vi "OFDM_demo.vi"() -> ()   [LabVIEW 2009]
uses:
  <vilib>/imath/engines/lvmath2/RunTimeEngine/ErrorHandling/NIMS_Finalize Error.vi
  <vilib>/imath/engines/lvmath2/RunTimeEngine/Parser/MC_Version.vi
  <vilib>/imath/engines/lvmath2/RunTimeEngine/NodeEndStatement/NIMS_NodeEndStatement_Output.vi
  <instcachedir>/0/NIMS_NodeEndStatement_Output_53EC0D466D134D7ABD903AC30B43404B.lvgen/NIMS_NodeEndStatement_Output_53EC0D466D134D7ABD903AC30B43404B_001.vi
  <vilib>/imath/engines/lvmath2/RunTimeEngine/RangeToken/NIMS_Range.vi
  <instcachedir>/0/NIMS_Range_08574DECC23E450FAF0AC0BC39E6BEA7.lvgen/NIMS_Range_08574DECC23E450FAF0AC0BC39E6BEA7_000.vi
  <vilib>/imath/engines/lvmath2/RunTimeEngine/BuiltInFunctions/round/NIMS_round(DBL-S).vi
  <vilib>/imathl/engines/lvmath/Functions/Error Handling/Create Error.vi
  <vilib>/imath/engines/lvmath/Functions/Error Handling/MC_Error Cluster From Error Code.vi
  <vilib>/imath/engines/lvmath2/RunTimeEngine/BuiltInFunctions/randnormal/NIMS_randnormal(1,I32).vi
  <vilib>/imath/engines/lvmath2/RunTimeEngine/RangeToken/NIMS_Range_R2 - Float.vi
  <instcachedir>/0/NIMS_Range_R2 - Float_93A1434467634702BCAD427B3499A8B4.lvgen/NIMS_Range_R2 - Float_93A1434467634702BCAD427B3499A8B4_000.vi
  <vilib>/imath/engines/lvmath/Functions/Error Handling/MergeErrorsWrapper.vi
  <vilib>/imath/engines/lvmath2/RunTimeEngine/ArithmeticOperatorToken/NIMS_ArithmeticOperator_plus.vi
  <instcachedir>/0/NIMS_ArithmeticOperator_plus_48B9519178ED42D7840F01273E784BFE.lvgen/NIMS_ArithmeticOperator_plus_48B9519178ED42D7840F01273E784BFE_000.vi
  <vilib>/imath/engines/lvmath2/RunTimeEngine/CommandStatement/MC_CommandStatement_break.vi
  <vilib>/imath/engines/lvmath2/RunTimeEngine/BuiltInFunctions/abs/NIMS_abs(signed).vi
  <instcachedir>/0/NIMS_abs(signed)_C4FCB8E6058B49B797C7C8D53CA5F6EC.lvgen/NIMS_abs(signed)_C4FCB8E6058B49B797C7C8D53CA5F6EC_000.vi
  <vilib>/imath/engines/lvmath2/RunTimeEngine/BuiltInFunctions/fft/NIMS_fft(GV).vi
  <instcachedir>/0/NIMS_fft(GV)_4C6467FC22F84E4BA42517A07EF978B0.lvgen/NIMS_fft(GV)_4C6467FC22F84E4BA42517A07EF978B0_001.vi
panel:
  in  "Number of Signals":dbl
  out "Frequency Domain":dbl[](graph)=[-65.85915777379863, -67.4159182508014, -83.98237928756325, -67.68454807939689, 0.001167659462857509, -62.00279471774978, -76.50031843632243, -79.84930333750974, -0.002321301830740114, -70.28161681379156, -75.37014688475936, -71.43223279356836, 0.0019758076165627735, -67.19023864671585, -59.326071900571705, -71.57758360782793, -0.0033451837990704854, -64.73231439603472, -68.3545781993946, -64.47936727351482, -0.004934079437755126, -63.18690880959889, -76.85128578370852, -77.1128911079366, -0.0015364990671404202, -60.09670538205802, -70.0061247105409, -66.3416220582635, 0.00308476690655415, -65.11673413833363, -69.99982685419918, -70.73910551220207, -0.0003146063843862787, -74.23065363786773, -82.56015032934161, -73.17243303091855, -0.005390191213401431, -64.32159403220355, -71.98817626923424, -69.2227375887466, -0.0025172993098405987, -66.25303750066834, -71.07288503298095, -68.5714475641465, -0.0026506959056577543, -72.79019967143984, -67.38892881214208, -63.8704912590564, 0.00015780098831987704, -68.67653217007089, -64.72051278103325, -64.4623299664106, 0.002984864272674666, -68.607590443405, -63.48155974398481, -66.18996423364395, -0.0027916165109335765, -63.627998158951996, -66.10830696818293, -71.77885901545312, -0.005305794062812742, -68.5330696250455, -65.18053285890313, -75.28656898448178, -0.0012317224408319144, -66.48761574232225, -65.79637197270438, -66.5523728488871, -0.002458779881879369, -64.93250339047772, -66.95401625552422, -72.71143622458413, -0.003663998535422267, -74.4964256353411, -71.53601578586682, -72.10926464858508, -0.0033669659636299397, -81.08779383955226, -69.63851872055983, -66.00644993381869, 0.002853851739313183, -65.03887110061628, -71.65894945859802, -68.7667431871805, 0.001286174703623317, -64.82909545506283, -67.84252983844794, -64.00457445122368, -0.0005370860401690884, -68.57259285794203, -73.0607979439583, -67.38041679413246, -0.000819699000330847, -71.11688188519892, -79.12328832965329, -74.4243659108799, -0.003680712718152329, -66.39506517793357, -72.10292803376697, -73.75934014796238, -0.0012648503306429636, -75.48974485549587, -67.35819567344844, -66.29114964266908, 0.0011096917850492642, -75.78825076994536, -68.6498880937598, -73.89622602097464, 0.00450716809119083, -70.98318173363074, -71.3103499892423, -73.81175836011673, -0.001276663889058421, -64.46629884383417, -74.36488154213885, -67.93429426887408, 0.0033684081216353097, -77.79388616517662, -66.26157587608216, -72.76220739766408, -0.0005132127073009369, -70.04594038061202, -73.19573222166245, -67.47769079029007, 0.0005524955358213877, -77.54300550351729, -71.04328528942425, -76.2420773706609, 6.0177378814099844, -76.2420773706609, -71.04328528942425, -77.54300550351729, 0.0005524955358213877, -67.47769079029007, -73.19573222166245, -70.04594038061202, -0.0005132127073009369, -72.76220739766408, -66.26157587608216, -77.79388616517662, 0.0033684081216353097, -67.93429426887408, -74.36488154213885, -64.46629884383417, -0.001276663889058421, -73.81175836011673, -71.3103499892423, -70.98318173363074, 0.00450716809119083, -73.89622602097464, -68.6498880937598, -75.78825076994536, 0.0011096917850492642, -66.29114964266908, -67.35819567344844, -75.48974485549587, -0.0012648503306429636, -73.75934014796238, -72.10292803376697, -66.39506517793357, -0.003680712718152329, -74.4243659108799, -79.12328832965329, -71.11688188519892, -0.000819699000330847, -67.38041679413246, -73.0607979439583, -68.57259285794203, -0.0005370860401690884, -64.00457445122368, -67.84252983844794, -64.82909545506283, 0.001286174703623317, -68.7667431871805, -71.65894945859802, -65.03887110061628, 0.002853851739313183, -66.00644993381869, -69.63851872055983, -81.08779383955226, -0.0033669659636299397, -72.10926464858508, -71.53601578586682, -74.4964256353411, -0.003663998535422267, -72.71143622458413, -66.95401625552422, -64.93250339047772, -0.002458779881879369, -66.5523728488871, -65.79637197270438, -66.48761574232225, -0.0012317224408319144, -75.28656898448178, -65.18053285890313, -68.5330696250455, -0.005305794062812742, -71.77885901545312, -66.10830696818293, -63.627998158951996, -0.0027916165109335765, -66.18996423364395, -63.48155974398481, -68.607590443405, 0.002984864272674666, -64.4623299664106, -64.72051278103325, -68.67653217007089, 0.00015780098831987704, -63.8704912590564, -67.38892881214208, -72.79019967143984, -0.0026506959056577543, -68.5714475641465, -71.07288503298095, -66.25303750066834, -0.0025172993098405987, -69.2227375887466, -71.98817626923424, -64.32159403220355, -0.005390191213401431, -73.17243303091855, -82.56015032934161, -74.23065363786773, -0.0003146063843862787, -70.73910551220207, -69.99982685419918, -65.11673413833363, 0.00308476690655415, -66.3416220582635, -70.0061247105409, -60.09670538205802, -0.0015364990671404202, -77.1128911079366, -76.85128578370852, -63.18690880959889, -0.004934079437755126, -64.47936727351482, -68.3545781993946, -64.73231439603472, -0.0033451837990704854, -71.57758360782793, -59.326071900571705, -67.19023864671585, 0.0019758076165627735, -71.43223279356836, -75.37014688475936, -70.28161681379156, -0.002321301830740114, -79.84930333750974, -76.50031843632243, -62.00279471774978, 0.001167659462857509, -67.68454807939689, -83.98237928756325, -67.4159182508014]
  out "Time Domain":dbl[](graph)=[32.00017112657278, -0.9983639293211752, 0.0008735355765997774, -1.0006091864923676, -0.0008656869615855403, -1.0002335780936629, -0.00012129659837191426, -1.0001721698210528, -0.005885422759168148, -0.995466661227796, -0.004419503619924629, -0.9948777723809261, 0.009332716893097842, -1.0031621642565403, -0.005016797304348691, -0.9964860889351613, -0.0021928490793982924, -1.0024576825906244, -0.006738884366811255, -0.9987835275908614, 0.0039564770633647, -1.0003854961966576, 6.529678604641038e-06, -0.9970424913742466, 0.003502863458182443, -1.000692082391001, 0.0016250124608794567, -0.99422494631012, 0.003640914889297361, -0.9998432185664662, -0.0005447667660256039, -0.996443898165778, 0.0003257808711581042, -0.9996152464607571, -0.002224165093202351, -0.9978196895746773, -0.006961344911486943, -1.0056132621276692, 0.0035615820280402053, -0.9984954841944591, 0.0023471787616144947, -1.0003846450004907, 0.0003302196259483037, -0.9990707669254306, 0.0036869433448601186, -0.9959639631261131, -0.0024015922345509873, -0.9990241319338568, -0.0014280381465069918, -0.9992900557634233, -0.0006415258476339477, -1.0039434357240529, -0.003933601587931967, -1.0019313163574013, 0.0005454145473986448, -1.0018604304189782, 0.00403129748804911, -0.995437793641305, -0.005078931896044563, -1.0004495062228045, -0.005667783175749135, -0.9950542453227285, -0.0010337477168682106, -1.0022702517624842, 31.996027861003995, -0.9992514696156752, 0.0023767417816136084, -0.9997573290965603, -0.00039079003427221735, -0.9972134852336257, 0.005253686163457493, -1.0019939747139937, -0.004615533899253865, -0.9999051627019617, 0.00174799695255463, -1.0008786334695843, 0.001040669585266476, -1.005631026866133, -0.00547826317021149, -1.0023984346670276, -0.0027209500680011023, -0.996926210417798, 0.004245827029374424, -0.9908809690660855, 0.0012736112257591991, -0.9983506650129511, -0.0024325566434215723, -1.0006700170865472, 0.003758930557249231, -1.0008199390652954, -0.00495900637739975, -1.003195189844263, -0.003449946260355973, -1.0008844588828651, -0.004112811651621141, -0.9995692117684838, 0.00039901886682617096, -1.000092063923351, 0.0021904132853824945, -0.9996356218624468, -0.0031081899271052653, -0.9991290221268253, 0.0027814082328749845, -1.0042300825504513, 0.0007163755121893314, -1.0013738837926813, -0.002538792067750837, -0.9997340068007473, 0.0031145063355714833, -1.00265950628907, -0.0004994034431624302, -0.9953760542096003, -0.002220859056506546, -1.0028537088428187, -0.0012009398756833648, -0.9963876808995135, 0.004768760241834631, -0.9988748054848854, 0.0004629995822051019, -0.9931078961670632, 0.002545476360266715, -1.0019962837613938, -0.0022606422179376326, -0.9955786638603721, -0.0006924783241974094, -1.0028097946283656, 0.0022509910529535946, -1.0043067841099833, 31.99308003375583, -1.0001975340020772, 0.0021521854173844873, -0.9964118152399534, 0.003451367454775092, -0.9982888588698008, 0.006709484384478659, -0.9943155486316583, 0.0023814148373482464, -0.9979859342389567, 0.002235599312541466, -1.0029388948536755, -0.0020749778600156654, -1.0046658275230822, -0.0076258112996254925, -0.9963324978398147, 0.007018563793711626, -0.9988749930014421, 0.00419471946131488, -0.997885450006954, -0.000586527863609928, -1.0024712482193048, -0.00031637483178920025, -1.0025777139206555, -0.001953463813398981, -1.0035333596290277, 0.0023257692492336048, -1.001220034251286, 0.001257832921962865, -1.0066843368331628, -0.004167328879506316, -0.9968152695189401, -0.004023488352167673, -1.0010141187149342, -0.007793457377208724, -0.9939375030812706, 0.002679938909838572, -1.0030008921892934, -0.0027638335569222555, -0.9954753924483939, -0.0003532745138856433, -0.9989481095190874, 0.005446015647737861, -0.9990239921663309, 9.144118346675314e-05, -0.9954959687509111, 0.0016108315870509322, -1.001295057213418, 0.003976438371584, -0.9974036072176263, -0.0015846434345923427, -0.9988861699074967, -0.003392541800487504, -0.9982390802100563, 0.0036750752995973156, -0.995471791777558, -0.006357595250655916, -0.9961930030453976, 0.006218886482116794, -0.9963854116294458, 0.0015459424890115557, -1.0002871409447218, 0.004653758434292616, -0.9969379199508, 31.998048597308518, -1.0035594998638433, 0.0030963177265235426, -0.9950825134768049, 0.004802706036061261, -0.9992790390451182, -0.003243995550517567, -1.0004121110728081, -0.0048345104142916324, -0.9974509412817338, -0.0008401960332384194, -1.0026873100338278, -0.001812520478654137, -0.9995563589014098, 0.006353744263335169, -0.9958356652642084, -0.00061226910175056, -0.999903912003857, -0.0022882196239423047, -0.9954445218993866, 0.0028368358149186636, -1.00261683845596, -0.002908757012912921, -0.9995071294372216, 0.000414888488207161, -0.9969790517863687, -0.0008200011831270629, -1.0013262295799326, -0.002067682657645524, -0.9987383371128324, -0.003963659283908664, -0.9997287880169212, -0.0026884880643222673, -0.9989105592767628, 0.005312504036034002, -0.9985221726588239, 0.005200062201811754, -0.9963666307013581, 0.0015221330408544662, -0.9924922747698924, -0.0035005107429873336, -1.001262993368365, 0.002884221783838924, -1.0005058160650895, -0.0023166260464192374, -0.9996843969226641, 0.00119668421088456, -0.9994091827060291, 0.0030455085186469706, -0.9987931598804075, -0.0010070332858092136, -1.003742514286312, -0.004531225664429646, -0.9991358540649633, 0.009061211640491224, -0.9952836903142885, -5.751067806155039e-05, -1.0001578303184124, -0.0016500207627205188, -1.0031067884150275, -0.0030479446321801233, -1.0049642984334832, 7.883432739733821e-05, -1.0036481110726918]
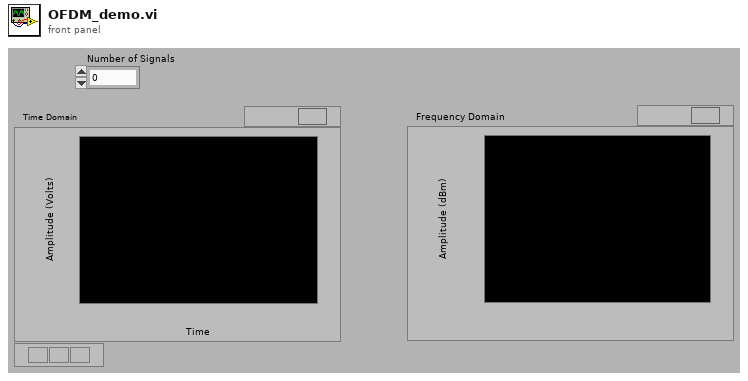
[diagram p1: front panel]
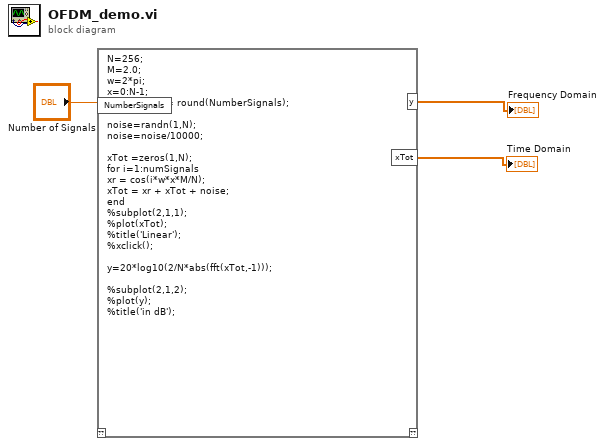
[diagram p0: block diagram]
diagram:
  n1 = mathscript code="N=256;\nM=2.0;\nw=2*pi;\nx=0:N-1;\nnumSignals = round(NumberSignals);\n\nnoise=randn(1,N);\nnoise=noise/10000;\n\nxTot =zeros(1,N);\nfor i=1:numSignals\nxr = cos(i*w*x*M/N);\nxTot = xr + xTot + noise;\nend\n%subplot(2,1,1);\n%plot(xTot);\n%title('Linear');\n%xclick();\n\ny=20*log10(2/N*abs(fft(xTot,-1)));\n\n%subplot(2,1,2);\n%plot(y);\n%title('in dB');"("NumberSignals"="Number of Signals") -> ("y"=→"Frequency Domain":dbl[], "xTot"=→"Time Domain":dbl[])  [unwired: 1 in, 1 out]
